vi "LINC Daemon Server.vi"(6 "instance":i32, 7 "timeout ms (1000)":i32=1000, 8 "port config":T1, 9 "port":u16, 10 "address":string, 11 "LINC session":refnum<class "LINC.lvclass">) -> ()   [LabVIEW 2018, in "STEPkgDriver_LINC.lvlib" / "LINC.lvclass"]
uses:
  LINC.lvclass
  LINC Global Session Mode.ctl
  STEPkgDriver_LINC.lvlib
  LINC Daemon Manager Mode.ctl
  LINC Port Config.ctl
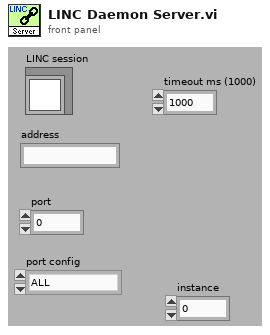
[diagram p1: front panel]
types:
  T1 = typedef "STEPkgDriver_LINC.lvlib/LINC Port Config.ctl" = enum16{"ALL", "CMD_ALL", "TLM_ALL", "TLM_BASIC"}
  T2 = typedef "STEPkgDriver_LINC.lvlib/LINC Daemon Manager Mode.ctl" = enum16{"INIT", "CLEAR", "GET"}
  T3 = typedef "STEPkgDriver_LINC.lvlib/LINC Global Session Mode.ctl" = enum16{"INIT", "CLEAR", "ADD_SESSION", "SET_CONNECTION", "SET_LISTENER", "SET_REFERENCE", "GET_SESSION"}
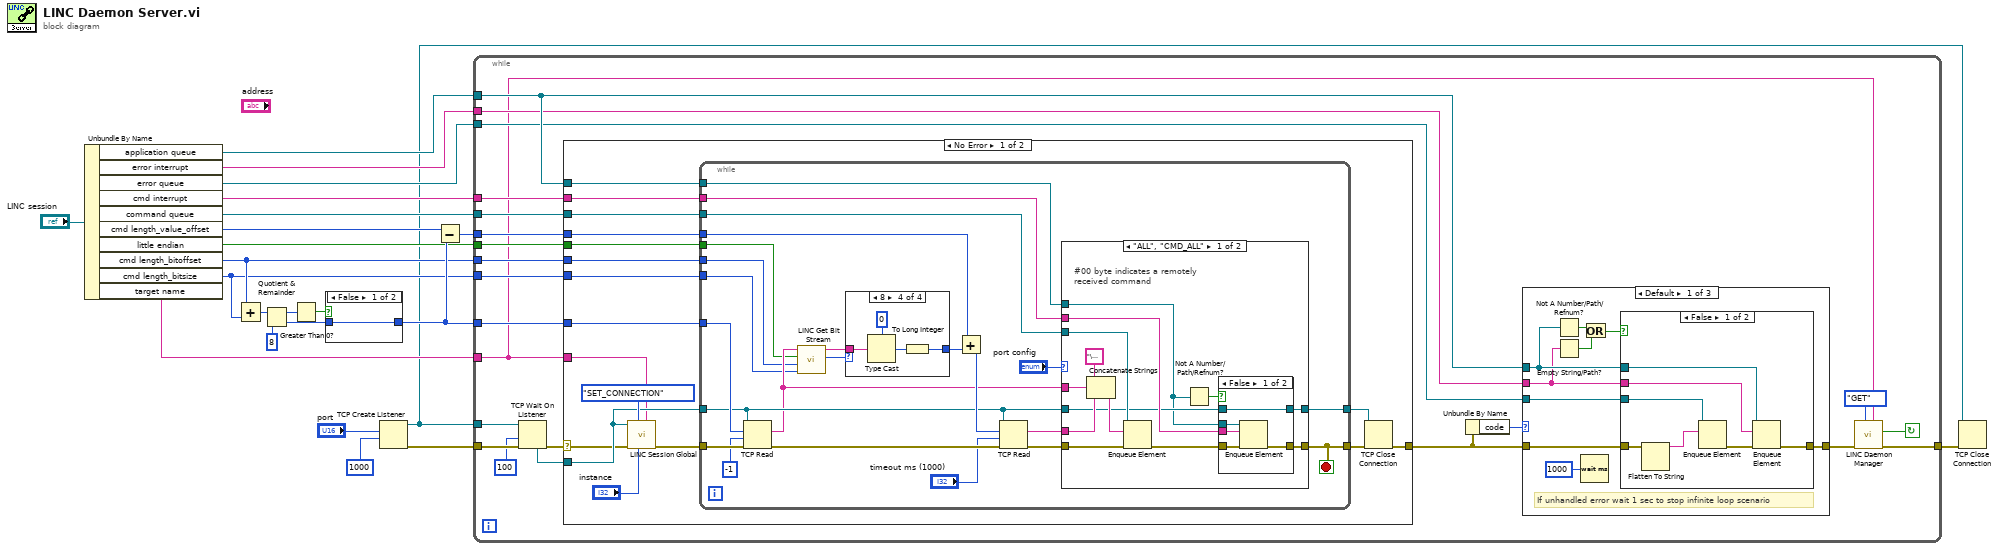
[diagram p0: block diagram]
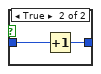
[diagram p2: hidden frame]
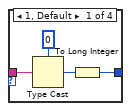
[diagram p5: hidden frame]
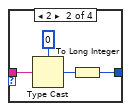
[diagram p6: hidden frame]
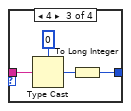
[diagram p7: hidden frame]
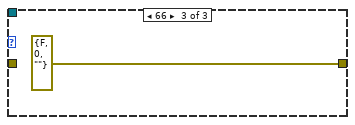
[diagram p11: hidden frame]
diagram:
  n1 = Unbundle By Name("LINC session") -> ("application queue"=w6:refnum<queue>, "error interrupt"=w7:string, "error queue"=w5:refnum<queue>, "cmd interrupt"=w14:string, "command queue"=w15:refnum<queue>, "cmd length_value_offset"=w21:i32, "little endian"=w8:bool, "cmd length_bitoffset"=w10:i32, "cmd length_bitsize"=w9:i32, "target name"=w11:string)
  n2 = Add(x=w10, y=w9) -> (x+y=w23:i32)
  n3 = Quotient & Remainder(x=w23, y=8) -> (x-y*floor(x/y)=w20:i32, floor(x/y)=w18:i32)
  n4 = Greater Than 0?(x=w20) -> (x > 0?=w19:bool)
  n5 = case shown="False" w19 {
    tunnel: w18 -> [w24 w26]
    tunnel: [w24 w25] -> w16
    frame False {
    }
    frame True {
      n6 = Increment(x=w26) -> (x+1=w25:i32)
    }
  }
  n7 = TCP Create Listener(9:1000 ("timeout ms (25000)"), 10:"port") -> (0:w1:errorcluster, 3:w2:refnum<k5>)  [unwired: 1 in, 3 out]
  n8 = Subtract(x=w21, y=w16) -> (x-y=w17:i32)
  n9 = while {
    tunnel: w16 -> [w42]
    tunnel: w11 -> [w27]
    tunnel: w1 -> [w47]
    tunnel: w17 -> [w43]
    tunnel: w15 -> [w46]
    tunnel: w6 -> [w37]
    tunnel: w14 -> [w45]
    tunnel: w2 -> [w44]
    tunnel: w10 -> [w40]
    tunnel: w9 -> [w39]
    tunnel: w8 -> [w38]
    tunnel: w7 -> [w36]
    tunnel: w5 -> [w35]
    tunnel: [w30] -> w3
    stop <- w29 continue-if-true
    n10 = TCP Wait On Listener(8:w47, 9:100 ("timeout ms (wait forever: -1)"), 11:w44) -> (0:w32:errorcluster, 4:w41:refnum<k5>)  [unwired: 4 out]
    n11 = case shown="No Error" w32 {
      selector: w32 -> [w50 _]
      tunnel: w46 -> [w65 _]
      tunnel: w45 -> [w64 _]
      tunnel: w43 -> [w61 _]
      tunnel: w42 -> [w60 _]
      tunnel: w41 -> [w58 _]
      tunnel: w40 -> [w57 _]
      tunnel: w39 -> [w56 _]
      tunnel: w38 -> [w55 _]
      tunnel: w37 -> [w54 _]
      tunnel: w27 -> [w53 _]
      tunnel: [w52 _] -> w34
      frame No Error {
        n12 = call "LINC Session Global.vi"("target name"=w53, "value in"="instance", "mode"=LINC_Global_Session_Mode."SET_CONNECTION", "error in (no error)"=w50, "connection in"=w58) -> ("error out"=w51:errorcluster)  [unwired: 2 in, 4 out]
        n13 = while {
          tunnel: w51 -> [w88]
          tunnel: w58 -> [w78]
          tunnel: [w68] -> w63
          tunnel: w60 -> [w83]
          tunnel: w61 -> [w82]
          tunnel: w65 -> [w80]
          tunnel: w54 -> [w69]
          tunnel: w64 -> [w79]
          tunnel: [w77] -> w62
          tunnel: w57 -> [w73]
          tunnel: w56 -> [w72]
          tunnel: w55 -> [w70]
          stop <- w68 stop-if-true
          n14 = TCP Read(connection ID=w78, bytes to read=w83, error in (no error)=w88, 9:-1 ("timeout ms (25000)")) -> (data out=w74:string, error out=w86:errorcluster)  [unwired: 2 out]
          n15 = call "LINC Get Bit Stream.vi"("bit size"=w72, "bit offset"=w73, "little endian"=w70, "data in"=w74) -> ("bytes"=w75:i32, "data out"=w76:string)  [unwired: 6 in]
          n16 = case shown="8" w75 {
            tunnel: w76 -> [w114 w118 w122 w126]
            tunnel: [w111 w115 w119 w123] -> w71
            frame 1, Default {
              n17 = Type Cast(type=u8 0, x=w114) -> (*(type *) &x=w112:u8)
              n18 = To Long Integer(number=w112) -> (32bit integer=w111:i32)
            }
            frame 2 {
              n19 = Type Cast(type=u16 0, x=w118) -> (*(type *) &x=w116:u16)
              n20 = To Long Integer(number=w116) -> (32bit integer=w115:i32)
            }
            frame 4 {
              n21 = Type Cast(type=u32 0, x=w122) -> (*(type *) &x=w120:u32)
              n22 = To Long Integer(number=w120) -> (32bit integer=w119:i32)
            }
            frame 8 {
              n23 = Type Cast(type=u64 0, x=w126) -> (*(type *) &x=w124:u64)
              n24 = To Long Integer(number=w124) -> (32bit integer=w123:i32)
            }
          }
          n25 = Add(x=w82, y=w71) -> (x+y=w81:i32)
          n26 = TCP Read(connection ID=w78, bytes to read=w81, error in (no error)=w86, 9:"timeout ms (1000)") -> (data out=w84:string, error out=w85:errorcluster)  [unwired: 2 out]
          n27 = case shown="\"ALL\", \"CMD_ALL\"" "port config" {
            tunnel: w85 -> [w101 w109]
            tunnel: w84 -> [w100 _]
            tunnel: w80 -> [w96 _]
            tunnel: w79 -> [w95 _]
            tunnel: w78 -> [w94 w110]
            tunnel: [w93 w110] -> w77
            tunnel: w74 -> [w91 _]
            tunnel: w69 -> [w90 _]
            tunnel: [w89 w109] -> w68
            frame "ALL", "CMD_ALL" {
              # "#00 byte indicates a remotely received command"
              n28 = Concatenate Strings("\u0000", w91, w100) -> (w99:string)
              n29 = Enqueue Element(queue=w96, element=w99, error in (no error)=w101) -> (error out=w98:errorcluster)  [unwired: 1 in, 2 out]
              n30 = Not A Number/Path/Refnum?(number/path/refnum=w90) -> (NaN/Path/Refnum?=w92:bool)
              n31 = case shown="False" w92 {
                tunnel: w98 -> [w106 w107]
                tunnel: [w105 w107] -> w89
                tunnel: w90 -> [w104 _]
                tunnel: w95 -> [w103 _]
                tunnel: w94 -> [w102 w108]
                tunnel: [w102 w108] -> w93
                frame False {
                  n32 = Enqueue Element(queue=w104, element=w103, error in (no error)=w106) -> (error out=w105:errorcluster)  [unwired: 1 in, 2 out]
                }
                frame True {
                }
              }
            }
            frame "TLM_ALL", "TLM_BASIC" {
            }
          }
        }
        n33 = TCP Close Connection(connection ID=w62, error in (no error)=w63) -> (error out=w52:errorcluster)  [unwired: 1 in, 1 out]
      }
      frame Error {
      }
    }
    n34 = Unbundle By Name(w34) -> ("code"=w48:i32)
    n35 = case shown="Default" w48 {
      tunnel: w34 -> [w130 w144 _]
      tunnel: [w129 w144 errorcluster {"status"=FALSE, "code"=0, "source"=""} ("error out")] -> w31
      tunnel: w37 -> [w133 _ _]
      tunnel: w36 -> [w132 _ _]
      tunnel: w35 -> [w128 _ _]
      frame Default {
        # "If unhandled error wait 1 sec to stop infinite loop scenario"
        n36 = Not A Number/Path/Refnum?(number/path/refnum=w133) -> (NaN/Path/Refnum?=w134:bool)
        n37 = Empty String/Path?(string/path=w132) -> (empty?=w135:bool)
        n38 = Wait (ms)(milliseconds to wait=u32 1000) -> ()  [unwired: 1 out]
        n39 = Or(x=w134, y=w135) -> (x .or. y?=w131:bool)
        n40 = case shown="False" w131 {
          tunnel: w133 -> [w142 _]
          tunnel: w132 -> [w141 _]
          tunnel: w130 -> [w139 w143]
          tunnel: [w140 w143] -> w129
          tunnel: w128 -> [w136 _]
          frame False {
            n41 = Flatten To String(anything=w139) -> (data string=w137:string)  [unwired: 3 in, 2 out]
            n42 = Enqueue Element(queue=w136, element=w137) -> (error out=w138:errorcluster)  [unwired: 2 in, 2 out]
            n43 = Enqueue Element(queue=w142, element=w141, error in (no error)=w138) -> (error out=w140:errorcluster)  [unwired: 1 in, 2 out]
          }
          frame True {
          }
        }
      }
      frame 1 {
      }
      frame 66 {
      }
    }
    n44 = call "LINC Daemon Manager.vi"("target name"=w27, "mode"=LINC_Daemon_Manager_Mode."GET", "error in (no error)"=w31) -> ("error out"=w30:errorcluster, "running"=w29:bool)  [unwired: 7 in]
  }
  n45 = TCP Close Connection(connection ID=w2, error in (no error)=w3) -> ()  [unwired: 1 in, 2 out]
